vi "公式节点.vi"() -> ()   [LabVIEW 2010]
panel:
  out "y1":dbl format="%.2f"
  in  "n":dbl=3.0 format="%.2f"
  in  "m":dbl=2.0 format="%.2f"
  out "y":dbl format="%.2f"
  in  "x":dbl=4.0 format="%.2f"
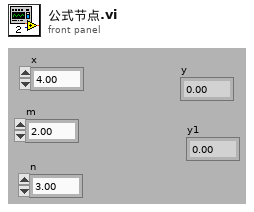
[diagram p1: front panel]
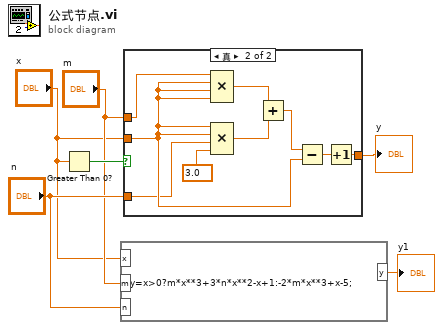
[diagram p0: block diagram]
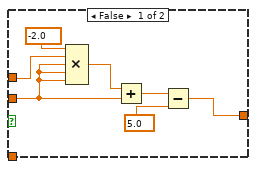
[diagram p2: hidden frame]
diagram:
  n1 = Greater Than 0?(x="x") -> (x > 0?=w6:bool)
  n2 = formula code="y=x>0?m*x**3+3*n*x**2-x+1:-2*m*x**3+x-5;"("x"="x", "m"="m", "n"="n") -> ("y"=→"y1":dbl)
  n3 = case shown="真" w6 {
    tunnel: "x" -> [w10 w19]
    tunnel: [w7 w21] -> w5
    tunnel: "m" -> [w13 w20]
    tunnel: "n" -> [_ w18]
    frame False {
      n4 = Compound Arithmetic op=MULTIPLY(-2.0 ("value"), w13, w10, w10, w10) -> (w11:dbl)
      n5 = Add(x=w11, y=w10) -> (x+y=w8:dbl)
      n6 = Subtract(x=w8, y=5.0) -> (x-y=w7:dbl)
    }
    frame True {
      n7 = Compound Arithmetic op=MULTIPLY(w20, w19, w19, w19) -> (w16:dbl)
      n8 = Compound Arithmetic op=MULTIPLY(w19, w19, w18, 3.0 ("y")) -> (w15:dbl)
      n9 = Add(x=w16, y=w15) -> (x+y=w14:dbl)
      n10 = Subtract(x=w14, y=w19) -> (x-y=w22:dbl)
      n11 = Increment(x=w22) -> (x+1=w21:dbl)
    }
  }
  "y" <- w5
